vi "Write Actor.vi"(7 "Actor in":refnum<data-value>, 10 "Actor":refnum<data-value>) -> (5 "Actor out":refnum<data-value>)   [LabVIEW 2020, in "jettl.lvlib"]
uses:
  jettl.lvlib
  Actor/Actor.lvclass
  Msg/Msg.lvclass
  Msgs.ctl
  Layer.ctl
  Refs/Refs.lvclass
  Actor.ctl
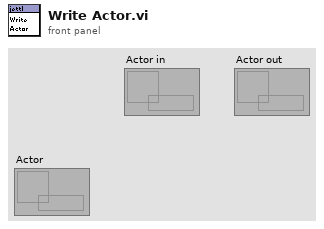
[diagram p1: front panel]
types:
  T1 = typedef "jettl.lvlib/Actor.ctl" = cluster{"Layer":T2, "Actor":refnum<class "Actor.lvclass">, "Refs":refnum<class "Refs.lvclass">}
  T2 = typedef "jettl.lvlib/Layer.ctl" = cluster{"Msgs":T3, "Leaf":bool, "Index":i32}
  T3 = typedef "jettl.lvlib/Msgs.ctl" = set{refnum<class "Msg.lvclass">}
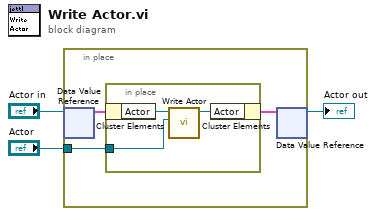
[diagram p0: block diagram]
diagram:
  n1 = in-place {
    in-place-border: "Actor" -> [w4]
    n2 = in-place-dvr #1("Actor in") -> (w6:T1)  [unwired: 1 out]
    n3 = in-place {
      in-place-border: w4 -> [w7]
      n4 = in-place-cluster #2(w6) -> ("Actor"=w9:refnum<class "Actor.lvclass">)
      n5 = call-dynamic "Write Actor.vi"("Actor"=w7, "Actor in"=w9) -> ("Actor out"=w8:refnum<class "Actor.lvclass">)  [unwired: 9 in]
      n6 = in-place-cluster #2("Actor"=w8) -> (w5:T1)
    }
    n7 = in-place-dvr #1(w5) -> (→"Actor out":refnum<data-value>)  [unwired: 1 out]
  }
